vi "CR-字符图片显示.vi"(0 "Image in":T3(plugin-control), 5 "Font, Size & Style":T2={"Desired Font (Application)"=enum."User-specified Font", "[User-specified Font]"={"Font Name"="", "Size"=54, "Strikeout?"=FALSE, "Italic?"=FALSE, "Underline?"=FALSE, "Outline?"=FALSE, "Shadow?"=FALSE, "Bold?"=FALSE, "Rotation Angle"=0.0}, "Horizontal Alignment"=0, "Vertical Alignment"=0} {"Vertical Alignment" items=["Bottom", "Top", "Baseline"]; "Horizontal Alignment" items=["Left", "Center", "Right"]; "[User-specified Font]"."Rotation Angle" format="%.2f"}, 7 "是否检测到字符串":bool, 9 "String (OCR/OCV 1)":string, 11 "error in (no error)":errorcluster caption="错误输入（无错误）", 12 "ROI Descriptor":T1 {"Contours"."Type" items=["No Selection", "Point", "Line", "Rectangle", "Oval", "Polygon", "Freehand Region", "Annulus", "Unused2", "Unused3", "Broken Line", "Freehand Line", "Rotated Rectangle"]}) -> (4 "Image out":T3(plugin-control), 15 "error out":errorcluster caption="错误输出")   [LabVIEW 2017]
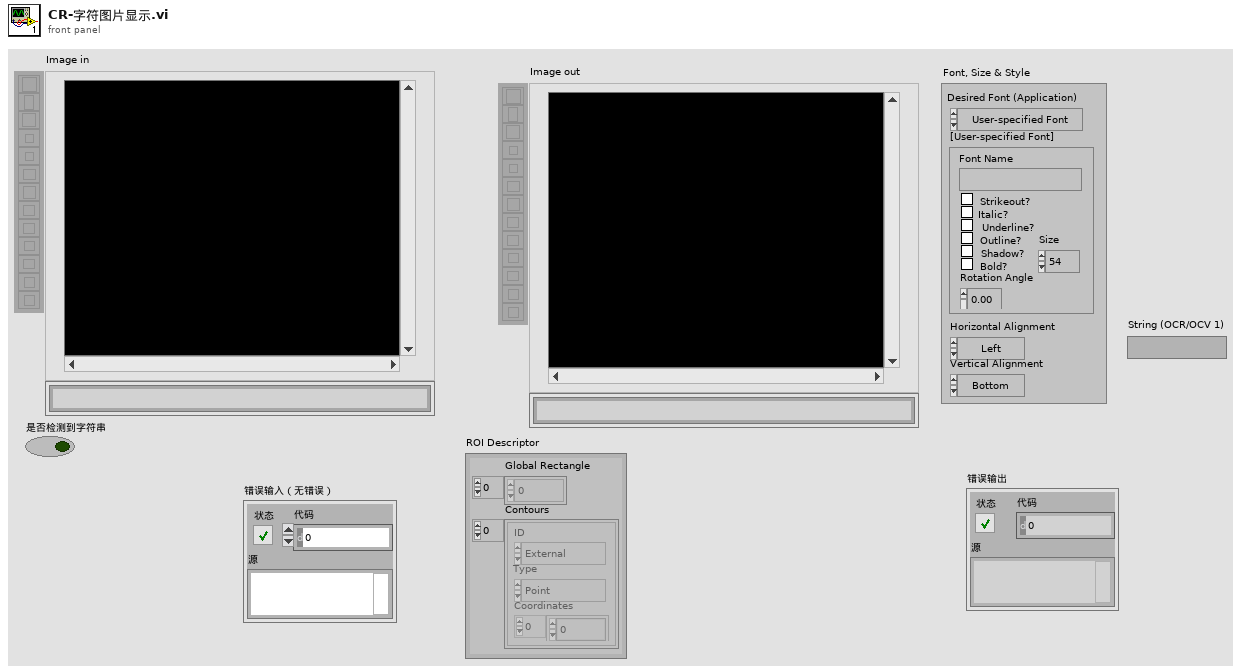
[diagram p1: front panel]
types:
  T1 = typedef "ROI Descriptor" = cluster{"Global Rectangle":i32[], "Contours":cluster{"ID":enum32{"External", "Internal"}, "Type":u32, "Coordinates":i32[]}[]}
  T2 = cluster{"Desired Font (Application)":enum16{"User-specified Font", "Application Font", "System Font", "Dialog Font"}, "[User-specified Font]":cluster{"Font Name":string, "Size":i16, "Strikeout?":bool, "Italic?":bool, "Underline?":bool, "Outline?":bool, "Shadow?":bool, "Bold?":bool, "Rotation Angle":dbl}, "Horizontal Alignment":i16, "Vertical Alignment":i16}
  T3 = typedef "IMAQ Image.ctl" = refnum<image>
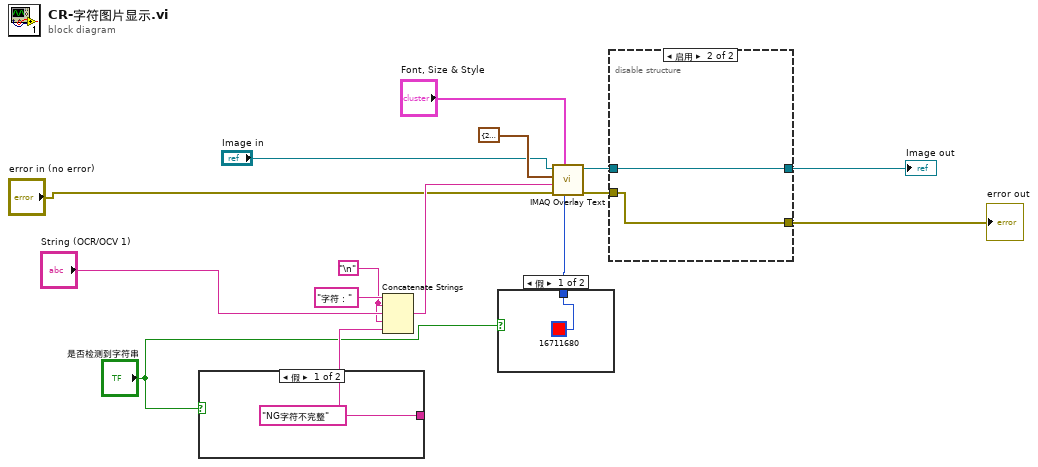
[diagram p0: block diagram]
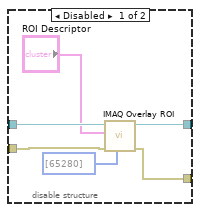
[diagram p2: hidden frame]
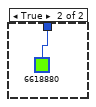
[diagram p3: hidden frame]
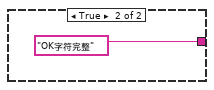
[diagram p4: hidden frame]
diagram:
  w8 = "\n"
  n1 = case shown="假" "是否检测到字符串" {
    tunnel: ["NG字符不完整" "OK字符完整"] -> w7
    frame False {
    }
    frame True {
    }
  }
  n2 = Concatenate Strings("字符：" ("字符串"), w8, "String (OCR/OCV 1)", w8, w7) -> (w15:string)
  n3 = case shown="假" "是否检测到字符串" {
    tunnel: [u32 16711680 ("Text Color (black)") u32 6618880 ("Text Color (black)")] -> w13
    frame False {
    }
    frame True {
    }
  }
  n4 = call "IMAQ Overlay Text"("Text Color (black)"=w13, "Font, Size & Style"="Font, Size & Style", "error in (no error)"="error in (no error)", "String"=w15, "Origin"=cluster{"X":i32, "Y":i32} {"X"=208, "Y"=232}, "Image"="Image in") -> ("error out"=w2:errorcluster, "Image Out"=w10:T3)  [unwired: 4 in]
  n5 = disable-structure shown="启用" {
    disable-tunnel: w10 -> [w25 w27]
    disable-tunnel: [w24 w27] -> w4
    disable-tunnel: w2 -> [w21 w26]
    disable-tunnel: [w20 w26] -> w1
    frame Disabled {
      n6 = call "IMAQ Overlay ROI"("Colors (Green)"=u32[] [65280], "error in (no error)"=w21, "ROI Descriptor"="ROI Descriptor", "Image"=w25) -> ("error out"=w20:errorcluster, "Image Out"=w24:T3)  [unwired: 6 in]
    }
    frame Enabled {
    }
  }
  "Image out" <- w4
  "error out" <- w1
